vi "Destroy.vi"(8 "error in (no error)":errorcluster, 11 "Serial Device in":refnum<class "Serial Device.lvclass">) -> (0 "error out":errorcluster)   [LabVIEW 2015, in "Serial Device.lvclass"]
uses:
  Serial Device.lvclass
  Serial Device.lvclass/Serial Device.ctl
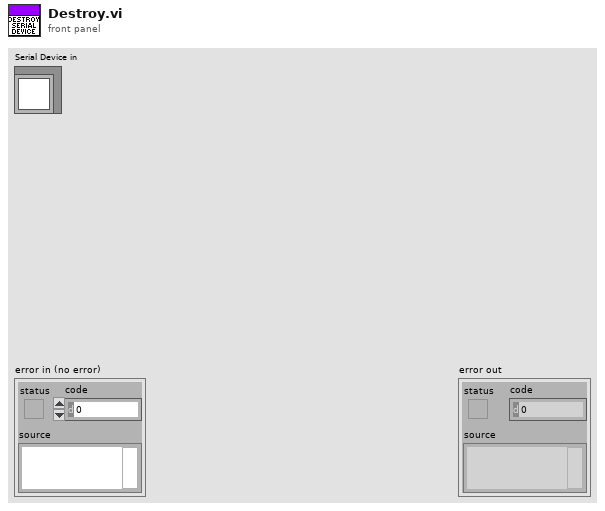
[diagram p1: front panel]
types:
  T1 = typedef "Semaphore RefNum" = refnum<k1>
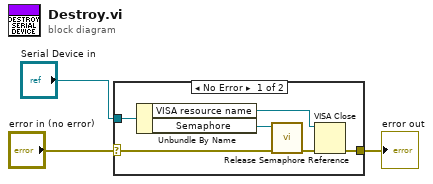
[diagram p0: block diagram]
diagram:
  n1 = case shown="No Error" "error in (no error)" {
    selector: "error in (no error)" -> [w6 w10]
    tunnel: [w4 w10] -> w2
    tunnel: "Serial Device in" -> [w9 _]
    frame No Error {
      n2 = Unbundle By Name(w9) -> ("VISA resource name"=w8:refnum<visa-resource-name>, "Semaphore"=w7:T1)
      n3 = call <vilib>:"Release Semaphore Reference.vi"("error in (no error)"=w6, "semaphore"=w7) -> ("error out"=w5:errorcluster)  [unwired: 8 in, 1 out]
      n4 = VISA Close(VISA resource name=w8, error in (no error)=w5) -> (error out=w4:errorcluster)
    }
    frame Error {
    }
  }
  "error out" <- w2
